vi "IP Address Facade.vi"(0 "Data In":T4 caption="数据输入", 2 "Display State In":T2={"Front Color"=1985280, "User Event"=refnum} caption="显示状态输入", 3 "Container State":T3 caption="容器状态") -> (6 "Data Out":T4 caption="数据输出", 7 "Display State Out":T2={"Front Color"=1985280, "User Event"=refnum} caption="显示状态输出", 8 "Action":T1 caption="动作")   [LabVIEW 2013, in "IP Adresss Control.xctl"]
uses:
  IP Adresss Control.xctl
  IP Address Data.ctl
  <vilib>/_xctls/Container State.ctl
  IP Address Status.ctl
  UserEvent/IP User Event.ctl
  <vilib>/_xctls/Action.ctl
  <vilib>/_xctls/XControlSupport.lvlib
panel:
  in  "IP3":u8
  in  "IP2":u8
  in  "IP1":u8
  in  "IP0":u8
  # "."
  # "."
  # "."
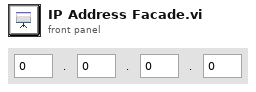
[diagram p1: front panel]
types:
  T1 = typedef "XControlSupport.lvlib/Action.ctl" = cluster{"Data Changed?":bool, "State Changed?":bool, "Action Name":string}
  T2 = typedef "IP Adresss Control.xctl/IP Address Status.ctl" = cluster{"Front Color":u32, "User Event":refnum<user-event>}
  T3 = typedef "XControlSupport.lvlib/Container State.ctl" = cluster{"Indicator?":bool, "Run Mode?":bool, " Refnum":refnum<vi>}
  T4 = typedef "IP Adresss Control.xctl/IP Address Data.ctl" = u32
  T5 = typedef "IP Adresss Control.xctl/IP User Event.ctl" = cluster{"Message":string}
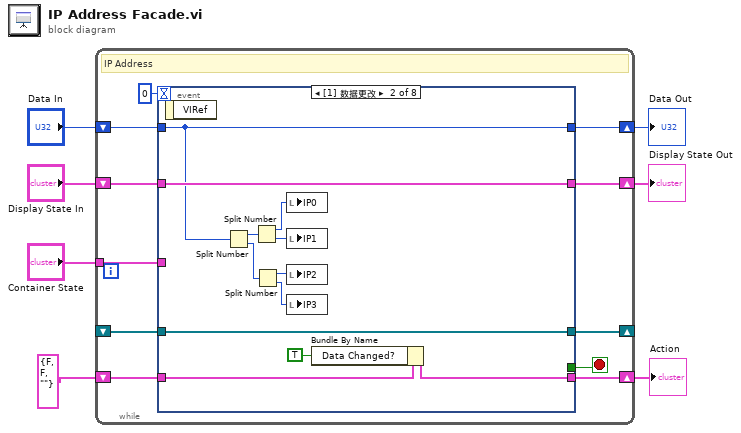
[diagram p0: block diagram]
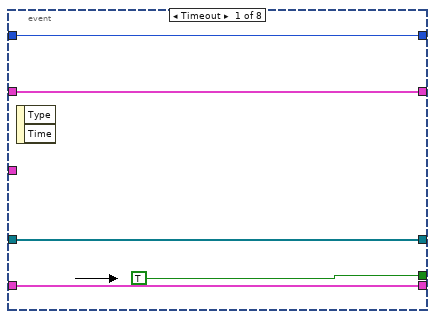
[diagram p2: hidden frame]
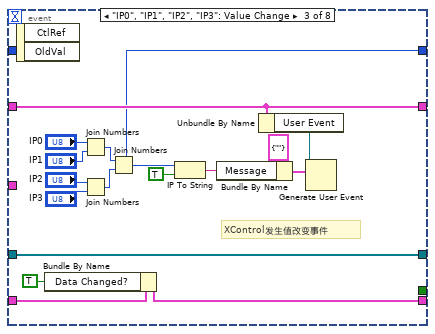
[diagram p3: hidden frame]
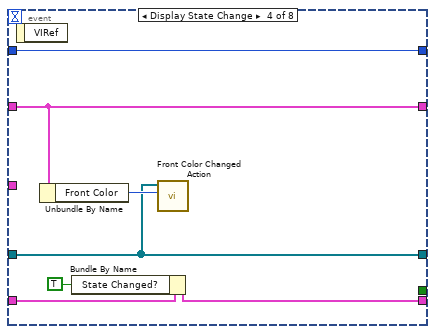
[diagram p4: hidden frame]
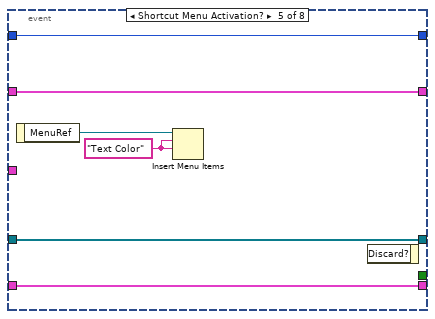
[diagram p5: hidden frame]
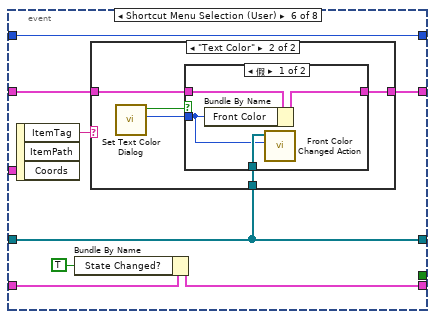
[diagram p6: hidden frame]
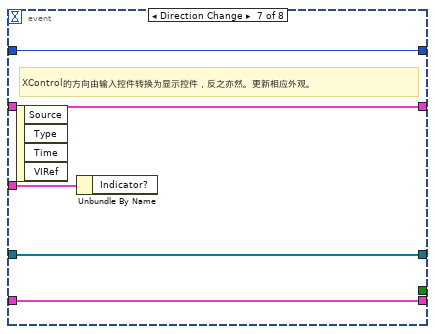
[diagram p9: hidden frame]
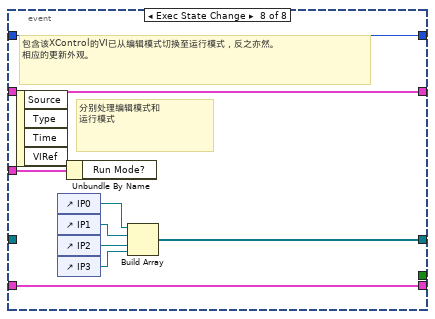
[diagram p10: hidden frame]
diagram:
  n1 = while {
    shift-right: [w17] -> w4
    shift-left: "Display State In" -> [w18]
    tunnel: "Container State" -> [w14]
    shift-right: [w12] -> w7
    shift-left: "Data In" -> [w13]
    shift-right: [w10] -> w2
    shift-left: T1 {"Data Changed?"=FALSE, "State Changed?"=FALSE, "Action Name"=""} ("Action") -> [w11]
    shift-right: [w9] -> _
    shift-left: _ -> [w8]
    stop <- w16 stop-if-true
    # "IP Address"
    n2 = event shown="[1] 数据更改" {
      selector: _ -> [_ _ _ _ _ _ _ _]
      dyn-events: _ -> [_ _ _ _ _ _ _ _]
      timeout: 0 -> [_ _ _ _ _ _ _ _]
      tunnel: w18 -> [w21 w35 w46 w58 w65 w72 w88 w97]
      tunnel: [w21 w35 w46 w58 w65 w71 w88 w97] -> w17
      tunnel: [TRUE _ _ _ _ _ _ _] -> w16
      tunnel: w14 -> [_ _ _ _ _ _ w89 w98]
      tunnel: w13 -> [w20 w34 _ w59 w64 w73 w87 w96]
      tunnel: [w20 w34 w44 w59 w64 w73 w87 w96] -> w12
      tunnel: [w22 w25 w37 w54 w63 w67 w86 w95] -> w10
      tunnel: w11 -> [w22 w27 w38 w57 w63 w69 w86 w95]
      tunnel: [w19 w26 w39 w55 w60 w68 w85 w90] -> w9
      tunnel: w8 -> [w19 w26 w39 w55 w60 w68 w85 _]
      event Timeout {
        n3 = event-data() -> ()  [unwired: 1 in, 2 out]
      }
      event Data Change {
        n4 = event-data() -> ()  [unwired: 1 in, 1 out]
        n5 = Split Number(x=w34) -> (hi(x)=w33:u16, lo(x)=w32:u16)
        n6 = Split Number(x=w33) -> (hi(x)=w31:u8, lo(x)=w30:u8)
        n7 = Split Number(x=w32) -> (hi(x)=w29:u8, lo(x)=w28:u8)
        n8 = local write "IP0"(w31) -> ()
        n9 = local write "IP1"(w30) -> ()
        n10 = local write "IP2"(w29) -> ()
        n11 = local write "IP3"(w28) -> ()
        n12 = Bundle By Name(cluster=w27, "Data Changed?"=TRUE) -> (w25:T1)
      }
      event "IP0", "IP1", "IP2", "IP3": Value Change {
        # "XControl发生值改变事件"
        n13 = event-data() -> ()  [unwired: 1 in, 2 out]
        n14 = Bundle By Name(cluster=w38, "Data Changed?"=TRUE) -> (w37:T1)
        n15 = Join Numbers(hi="IP0", lo="IP1") -> ((hi.lo)=w48:u16)
        n16 = Join Numbers(hi="IP2", lo="IP3") -> ((hi.lo)=w47:u16)
        n17 = Join Numbers(hi=w48, lo=w47) -> ((hi.lo)=w44:u32)
        n18 = IP To String(1:TRUE ("句点符号？(F)"), 2:w44) -> (0:w42:string)
        n19 = Bundle By Name(cluster=T5 {"Message"=""} ("事件数据"), "Message"=w42) -> (w40:T5)
        n20 = Unbundle By Name(w46) -> ("User Event"=w45:refnum<user-event>)
        n21 = Generate User Event(user event=w45, event data cluster=w40) -> ()  [unwired: 2 in, 2 out]
      }
      event Display State Change {
        n22 = event-data() -> ()  [unwired: 1 in, 1 out]
        n23 = Unbundle By Name(w58) -> ("Front Color"=w56:u32)
        n24 = Bundle By Name(cluster=w57, "State Changed?"=TRUE) -> (w54:T1)
        n25 = call "Front Color Changed Action.vi"("Color"=w56, "Control Ref"=w55) -> ()  [unwired: 9 in, 1 out]
      }
      event Shortcut Menu Activation? {
        w61 = "Text Color"
        n26 = event-data() -> ("MenuRef"=w62:refnum<k9>)  [unwired: 1 in]
        n27 = Insert Menu Items(7:w61, 8:w61, 9:w62) -> ()  [unwired: 3 in, 3 out]
        n28 = event-data() -> ()  [unwired: 2 in, 1 out]
      }
      event Shortcut Menu Selection (User) {
        n29 = event-data() -> ("ItemTag"=w70:string)  [unwired: 1 in, 2 out]
        n30 = Bundle By Name(cluster=w69, "State Changed?"=TRUE ("Data Changed?")) -> (w67:T1)
        n31 = case shown="\"Text Color\"" w70 {
          tunnel: w72 -> [w74 w78]
          tunnel: [w74 w77] -> w71
          tunnel: w68 -> [_ w76]
          frame "", Default {
          }
          frame "Text Color" {
            n32 = call "Set Text Color Dialog.vi"() -> ("Text Color Out"=w79:u32, "Cancelled?"=w75:bool)  [unwired: 10 in]
            n33 = case shown="假" w75 {
              tunnel: w79 -> [w80 _]
              tunnel: w78 -> [w83 w84]
              tunnel: [w82 w84] -> w77
              tunnel: w76 -> [w81 _]
              frame False {
                n34 = Bundle By Name(cluster=w83, "Front Color"=w80) -> (w82:T2)
                n35 = call "Front Color Changed Action.vi"("Color"=w80, "Control Ref"=w81) -> ()  [unwired: 9 in, 1 out]
              }
              frame True {
              }
            }
          }
        }
      }
      event Direction Change {
        # "XControl的方向由输入控件转换为显示控件，反之亦然。更新相应外观。"
        n36 = event-data() -> ()  [unwired: 1 in, 4 out]
        n37 = Unbundle By Name(w89) -> ()  [unwired: 1 out]
      }
      event Exec State Change {
        # "包含该XControl的VI已从编辑模式切换至运行模式，反之亦然。\n相应的更新外观。"
        # "分别处理编辑模式和\n运行模式"
        n38 = event-data() -> ()  [unwired: 1 in, 4 out]
        n39 = control-ref of="IP0"() -> (w91:refnum<vi>)
        n40 = control-ref of="IP1"() -> (w92:refnum<vi>)
        n41 = control-ref of="IP2"() -> (w93:refnum<vi>)
        n42 = control-ref of="IP3"() -> (w94:refnum<vi>)
        n43 = Unbundle By Name(w98) -> ()  [unwired: 1 out]
        n44 = Build Array(w91, w92, w93, w94) -> (w90:refnum<vi>[])
      }
    }
  }
  "Display State Out" <- w4
  "Data Out" <- w7
  "Action" <- w2
